vi "19-Match.vi"(10 "Base Orientation":T3, 11 "Sensor Orientations":T1(array[cluster])) -> (0 "max value":i32, 1 "Match Found?":bool, 2 "Match Info":T2, 3 "Orientation":T3)   [LabVIEW 2019, in "19.lvlib"]
uses:
  19.lvlib
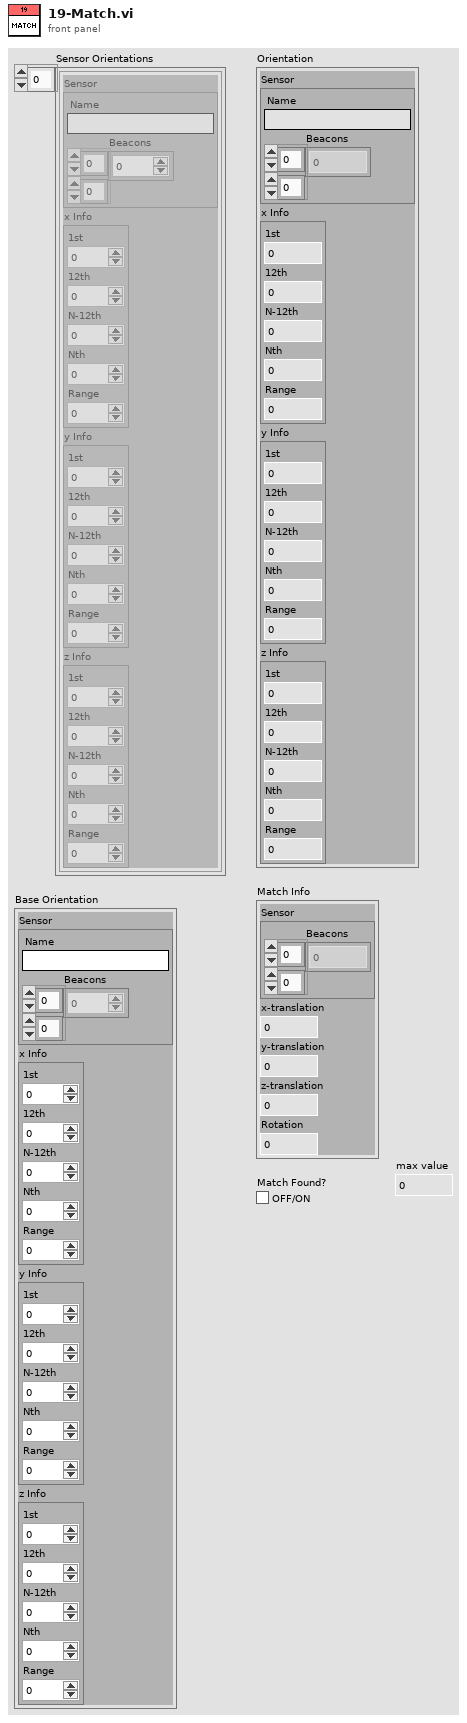
[diagram p1: front panel]
types:
  T1 = cluster{"Sensor":cluster{"Name":string, "Beacons":i32[][]}, "x Info":cluster{"1st":i32, "12th":i32, "N-12th":i32, "Nth":i32, "Range":i32}, "y Info":cluster{"1st":i32, "12th":i32, "N-12th":i32, "Nth":i32, "Range":i32}, "z Info":cluster{"1st":i32, "12th":i32, "N-12th":i32, "Nth":i32, "Range":i32}}[]
  T2 = cluster{"Sensor":cluster{"Beacons":i32[][]}, "x-translation":i32, "y-translation":i32, "z-translation":i32, "Rotation":i32}
  T3 = cluster{"Sensor":cluster{"Name":string, "Beacons":i32[][]}, "x Info":cluster{"1st":i32, "12th":i32, "N-12th":i32, "Nth":i32, "Range":i32}, "y Info":cluster{"1st":i32, "12th":i32, "N-12th":i32, "Nth":i32, "Range":i32}, "z Info":cluster{"1st":i32, "12th":i32, "N-12th":i32, "Nth":i32, "Range":i32}}
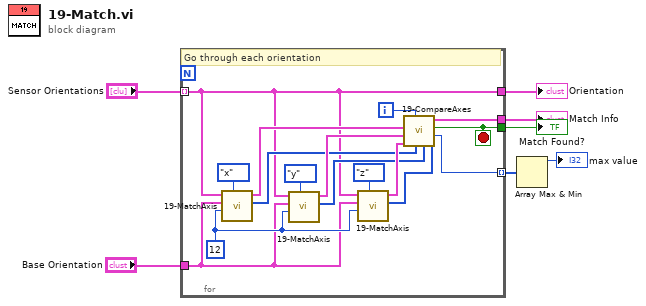
[diagram p0: block diagram]
diagram:
  n1 = for {
    tunnel: "Sensor Orientations" -> [w9] mode=indexing
    tunnel: [w19] -> w4
    tunnel: "Base Orientation" -> [w17]
    tunnel: [w18] -> w7
    tunnel: [w9] -> w6
    tunnel: [w8] -> w2 mode=indexing
    i -> [w10]
    stop <- w18 stop-if-true
    w20 = 12 ("Minimum Matches")
    # "Go through each orientation"
    n2 = call "19-MatchAxis.vi"("Axis"=enum16{"x", "y", "z"}."x", "Minimum Matches"=w20, "Base Sensor Orientation Info"=w17, "Orientation Info"=w9) -> ("Match Translations"=w13:i32[], "Matches"=w14:cluster{"Beacons":i32[][]}[])  [unwired: 6 in]
    n3 = call "19-MatchAxis.vi"("Axis"=enum16{"x", "y", "z"}."y", "Minimum Matches"=w20, "Base Sensor Orientation Info"=w17, "Orientation Info"=w9) -> ("Match Translations"=w12:i32[], "Matches"=w15:cluster{"Beacons":i32[][]}[])  [unwired: 6 in]
    n4 = call "19-MatchAxis.vi"("Axis"=enum16{"x", "y", "z"}."z", "Minimum Matches"=w20, "Base Sensor Orientation Info"=w17, "Orientation Info"=w9) -> ("Match Translations"=w11:i32[], "Matches"=w16:cluster{"Beacons":i32[][]}[])  [unwired: 6 in]
    n5 = call "19-CompareAxes.vi"("Match Translations z"=w11, "Match Translations y"=w12, "Match Translations x"=w13, "Rotation index"=w10, "Matches z"=w16, "Matches y"=w15, "Matches x"=w14) -> ("max value"=w8:i32, "Match Found?"=w18:bool, "Match Info"=w19:T2)  [unwired: 2 in]
  }
  "Match Found?" <- w7
  "Orientation" <- w6
  "Match Info" <- w4
  n6 = Array Max & Min(array=w2) -> (max value=→"max value":i32)  [unwired: 3 out]
